vi "DoubleArray2INIstring.vi"(4 "Array":dbl[](array[numeric])) -> (7 "String":string)   [LabVIEW 2013]
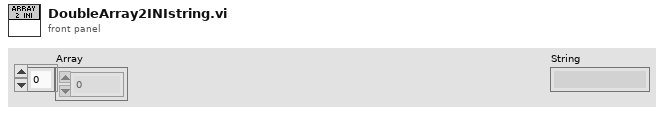
[diagram p1: front panel]
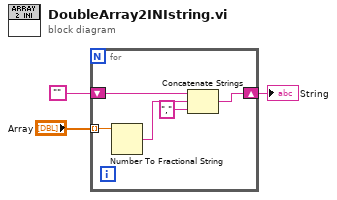
[diagram p0: block diagram]
diagram:
  n1 = for {
    tunnel: "Array" -> [w8] mode=indexing
    shift-right: [w5] -> w1
    shift-left: "" -> [w7]
    n2 = Number To Fractional String(number=w8) -> (F-format string=w6:string)  [unwired: 3 in]
    n3 = Concatenate Strings(w7, w6, ",") -> (w5:string)
  }
  "String" <- w1
